vi "Picolog Example Log Temp Fixed Interval.vi"() -> ()   [LabVIEW 2016]
uses:
  Controls/Thermocouple.ctl
  Controls/Temperature Units.ctl
  Controls/Fill Missing.ctl
  Controls/State Control.ctl
panel:
  in  "Tab Control":enum32{"Configuration", "Results"}(tab)
  in  "Thermocouples":T1[](array[typedef])=[107, 32, 32, 32, 32, 32, 32, 32, 32, 32] items=["B"=98, "E"=101, "J"=106, "K"=107, "N"=110, "R"=114, "S"=115, "T"=116, "Voltage"=120, "Internal"=0, "Off"=32]
  in  "Mains Frequency":i16(ring) items=["50 Hz", "60 Hz"]
  in  "Unit":T2
  in  "Sampling Interval [s]":dbl=0.2 min=0.1 max=100.0 step=0.1 format="%#_13g"
  in  "Fill Missing Points":T3 items=["QNaN", "Previous"]
  in  "Buffer Length":i32=128
  in  "Update Rate [s]":dbl=0.5
  out "Actual Interval [s]":dbl
  out "Error":errorcluster
  out "Temperature":waveform(dbl)[](graph)
  in  "Stop":bool
  # "PicoLog Thermocouple Demo"
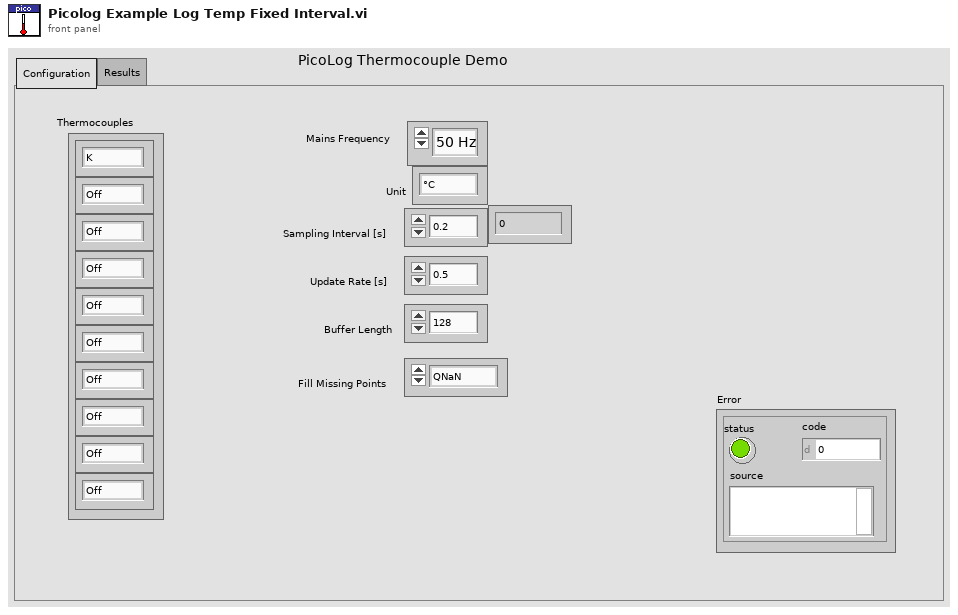
[diagram p1: front panel]
types:
  T1 = typedef "Thermocouple.ctl" = i8
  T2 = typedef "Temperature Units.ctl" = enum16{"°C", "°F", "K", "°R"}
  T3 = typedef "Fill Missing.ctl" = i16
  T4 = typedef "State Control.ctl" = enum16{"Initialize", "Idle", "Acquire", "Display", "Shutdown", "Quit", "Error"}
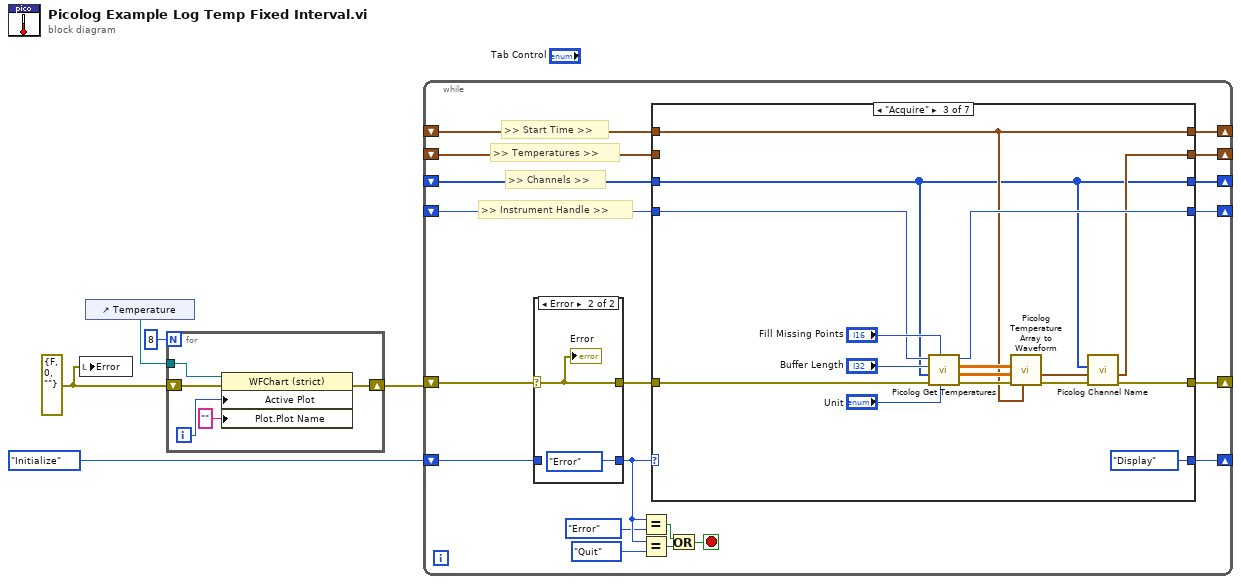
[diagram p0: block diagram]
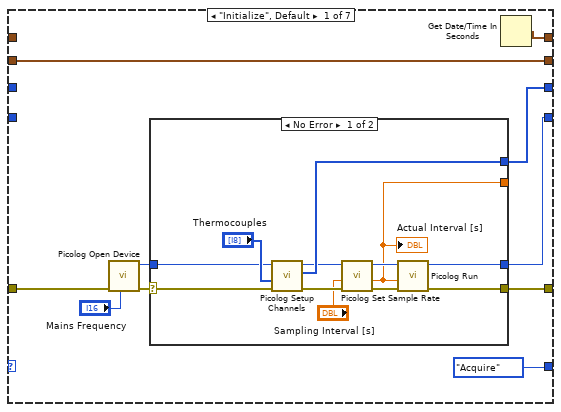
[diagram p3: hidden frame]
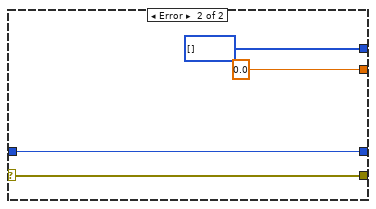
[diagram p4: hidden frame]
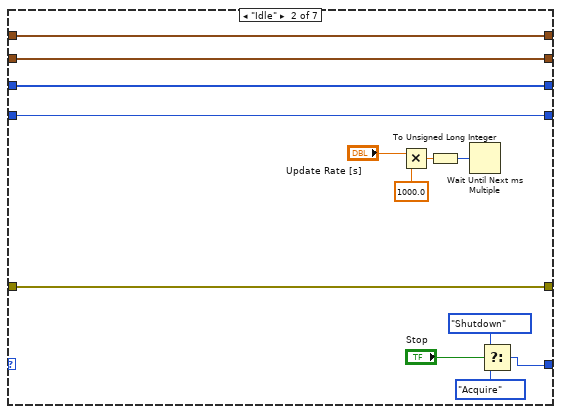
[diagram p5: hidden frame]
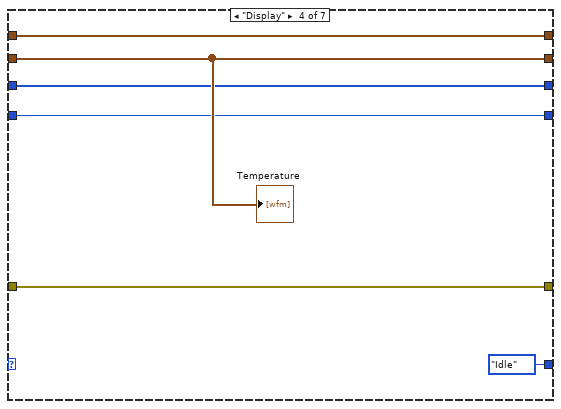
[diagram p6: hidden frame]
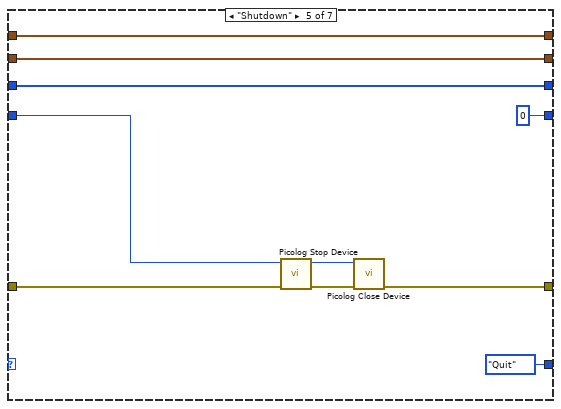
[diagram p7: hidden frame]
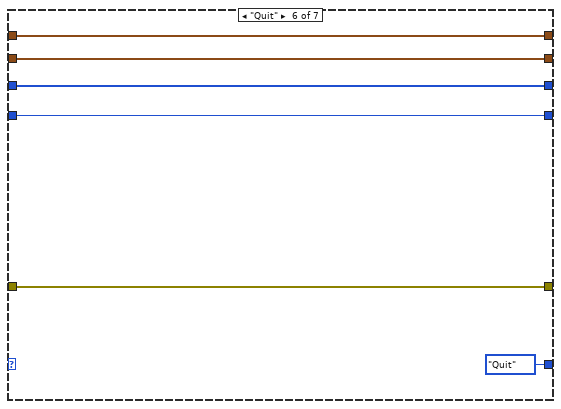
[diagram p8: hidden frame]
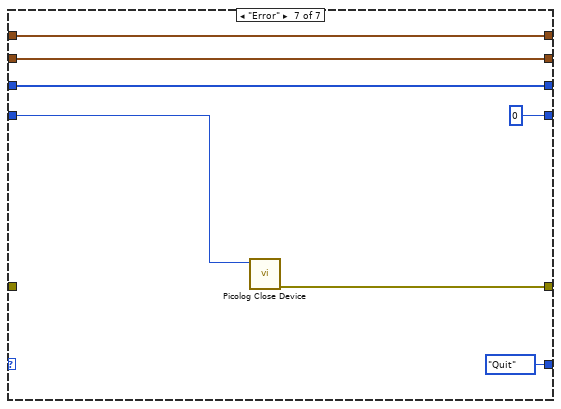
[diagram p9: hidden frame]
diagram:
  w3 = errorcluster {"status"=FALSE, "code"=0, "source"=""} ("Error Out")
  n1 = local write "Error"(w3) -> ()
  n2 = control-ref of="Temperature"() -> (w4:refnum<vi>)
  n3 = for {
    N: 8 -> [_]
    tunnel: w4 -> [w10]
    shift-right: [w8] -> w2
    shift-left: w3 -> [w9]
    i -> [w7]
    n4 = property class="WFChart (strict)"(reference=w10, error in=w9, "Active Plot"=w7, "Plot.Plot Name"="") -> (error out=w8:errorcluster)  [unwired: 1 out]
  }
  n5 = while {
    shift-right: [w20] -> _
    shift-left: _ -> [w28]
    shift-right: [w29] -> _
    shift-left: w2 -> [w13]
    shift-right: [w27] -> _
    shift-left: State_Control."Initialize" ("State") -> [w21]
    shift-right: [w26] -> _
    shift-left: _ -> [w25]
    shift-right: [w24] -> _
    shift-left: _ -> [w23]
    shift-right: [w12] -> _
    shift-left: _ -> [w11]
    stop <- w14 stop-if-true
    # ">> Start Time >>"
    # ">> Temperatures >>"
    # ">> Instrument Handle >>"
    # ">> Channels >>"
    n6 = case shown="Error" w13 {
      selector: w13 -> [w31 w32]
      tunnel: [w31 w32] -> w22
      tunnel: w21 -> [w30 _]
      tunnel: [w30 State_Control."Error" ("State")] -> w18
      frame No Error {
      }
      frame Error {
        "Error" <- w32
      }
    }
    n7 = Equal?(x=w18, y=State_Control."Error") -> (x = y?=w16:bool)
    n8 = Equal?(x=w18, y=State_Control."Quit") -> (x = y?=w15:bool)
    n9 = case shown="\"Acquire\"" w18 {
      tunnel: [w41 w72 w77 w92 i16 0 ("Instrument Handle Out") w106 i16 0 ("Instrument Handle Out")] -> w20
      tunnel: [w40 w71 w78 w91 w97 w107 w116] -> w29
      tunnel: w28 -> [_ w72 w79 w92 w103 w106 w117]
      tunnel: w22 -> [w39 w71 w80 w91 w104 w107 _]
      tunnel: [State_Control."Acquire" ("State") w69 State_Control."Display" ("State") State_Control."Idle" ("State") State_Control."Quit" ("State") State_Control."Quit" ("State") State_Control."Quit" ("State")] -> w27
      tunnel: [w37 w66 w76 w94 w102 w110 w113] -> w26
      tunnel: w25 -> [_ w66 w76 w94 w102 w110 w113]
      tunnel: [w36 w62 w74 w93 w100 w108 w114] -> w24
      tunnel: w23 -> [w36 w62 _ w93 w100 w108 w114]
      tunnel: [w34 w61 w73 w89 w95 w105 w111] -> w12
      tunnel: w11 -> [_ w61 w73 w89 w95 w105 w111]
      frame "Initialize", Default {
        n10 = call "Picolog Open Device.vi"("Mains Frequency"="Mains Frequency", "Error In"=w39) -> ("Error Out"=w35:errorcluster, "Instrument Handle Out"=w42:i16)  [unwired: 8 in]
        n11 = case shown="No Error" w35 {
          selector: w35 -> [w48 w59]
          tunnel: w42 -> [w51 w58]
          tunnel: [w50 w58] -> w41
          tunnel: [w49 w59] -> w40
          tunnel: [w44 0.0] -> _
          tunnel: [w47 i16[] [] ("Channels")] -> w34
          frame No Error {
            n12 = call "Picolog Setup Channels.vi"("Error In"=w48, "Configurations"="Thermocouples", "Instrument Handle"=w51) -> ("Error Out"=w53:errorcluster, "Channels"=w47:i16[], "Instrument Handle Out"=w46:i16)  [unwired: 6 in]
            n13 = call "Picolog Set Sample Rate.vi"("error in (no error)"=w53, "Sampling Interval [s]"="Sampling Interval [s]", "Instrument Handle In"=w46) -> ("error out"=w55:errorcluster, "Actual Sampling Interval [s]"=w44:dbl, "Instrument Handle Out"=w54:i16)  [unwired: 6 in]
            "Actual Interval [s]" <- w44
            n14 = call "Picolog Run.vi"("Error In"=w55, "Interval [s]"=w44, "Instrument Handle In"=w54) -> ("Error Out"=w49:errorcluster, "Instrument Handle Out"=w50:i16)  [unwired: 6 in, 1 out]
          }
          frame Error {
          }
        }
        n15 = Get Date/Time In Seconds() -> (seconds since 1Jan1904=w37:timestamp)
      }
      frame "Idle" {
        n16 = Multiply(x="Update Rate [s]", y=1000.0) -> (x*y=w64:dbl)
        n17 = To Unsigned Long Integer(number=w64) -> (unsigned 32bit integer=w63:u32)
        n18 = Wait Until Next ms Multiple(millisecond multiple=w63) -> ()  [unwired: 1 out]
        n19 = Select(t=State_Control."Shutdown" ("State"), s="Stop", f=State_Control."Acquire" ("State")) -> (s? t:f=w69:T4)
      }
      frame "Acquire" {
        n20 = call "Picolog Get Temperatures.vi"("Units"="Unit", "Fill Missing Points"="Fill Missing Points", "Error In"=w80, "Channels"=w73, "Buffer Length"="Buffer Length", "Instrument Handle In"=w79) -> ("Error Out"=w85:errorcluster, "Temperature"=w86:sgl[][], "Time [s]"=w87:dbl[][], "Instrument Handle Out"=w77:i16)  [unwired: 1 in, 1 out]
        n21 = call "Picolog Temperature Array to Waveform.vi"("Start Time"=w76, "Error In"=w85, "Temperatures"=w86, "Times [s]"=w87) -> ("Error Out"=w83:errorcluster, "Temperature Waveforms"=w84:waveform(dbl)[])  [unwired: 6 in]
        n22 = call "Picolog Channel Name.vi"("Error In"=w83, "Temperature Waveforms"=w84, "Channels"=w73) -> ("Error Out"=w78:errorcluster, "Temperature Waveforms with Names"=w74:waveform(dbl)[])  [unwired: 7 in]
      }
      frame "Display" {
        "Temperature" <- w93
      }
      frame "Shutdown" {
        n23 = call "Picolog Stop Device.vi"("Error In"=w104, "Instrument Handle In"=w103) -> ("Error Out"=w98:errorcluster, "Instrument Handle Out"=w99:i16)  [unwired: 8 in]
        n24 = call "Picolog Close Device.vi"("Error In"=w98, "Instrument Handle"=w99) -> ("Error Out"=w97:errorcluster)  [unwired: 9 in]
      }
      frame "Quit" {
      }
      frame "Error" {
        n25 = call "Picolog Close Device.vi"("Instrument Handle"=w117) -> ("Error Out"=w116:errorcluster)  [unwired: 10 in]
      }
    }
    n26 = Or(x=w16, y=w15) -> (x .or. y?=w14:bool)
  }
